vi "Main.vi"() -> ()   [LabVIEW 2015]
uses:
  TypeDefs/Queue Data.ctl
  FGV/Timer Actions.ctl
  SubVIs/App Data.vi
  SubVIs/App Strings.vi
panel:
  in  "Period [s]":dbl
  in  "Device name":tag="myDAQ1"
  out "Time Elapsed":dbl format="%<%M:%S>t"
  out "Status":string
  in  "Time [ms]":dbl
  in  "Frequency":dbl
  in  "Stop Button":bool
  in  "Acquire Button":bool
  out "Waveform Graph":dbl[](graph)
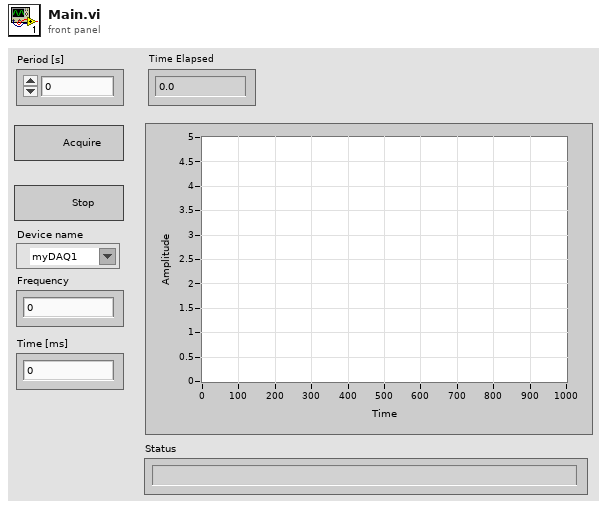
[diagram p1: front panel]
types:
  T1 = typedef "Timer Actions.ctl" = enum16{"Reset", "Get"}
  T2 = typedef "Queue Data.ctl" = cluster{"Action":string}
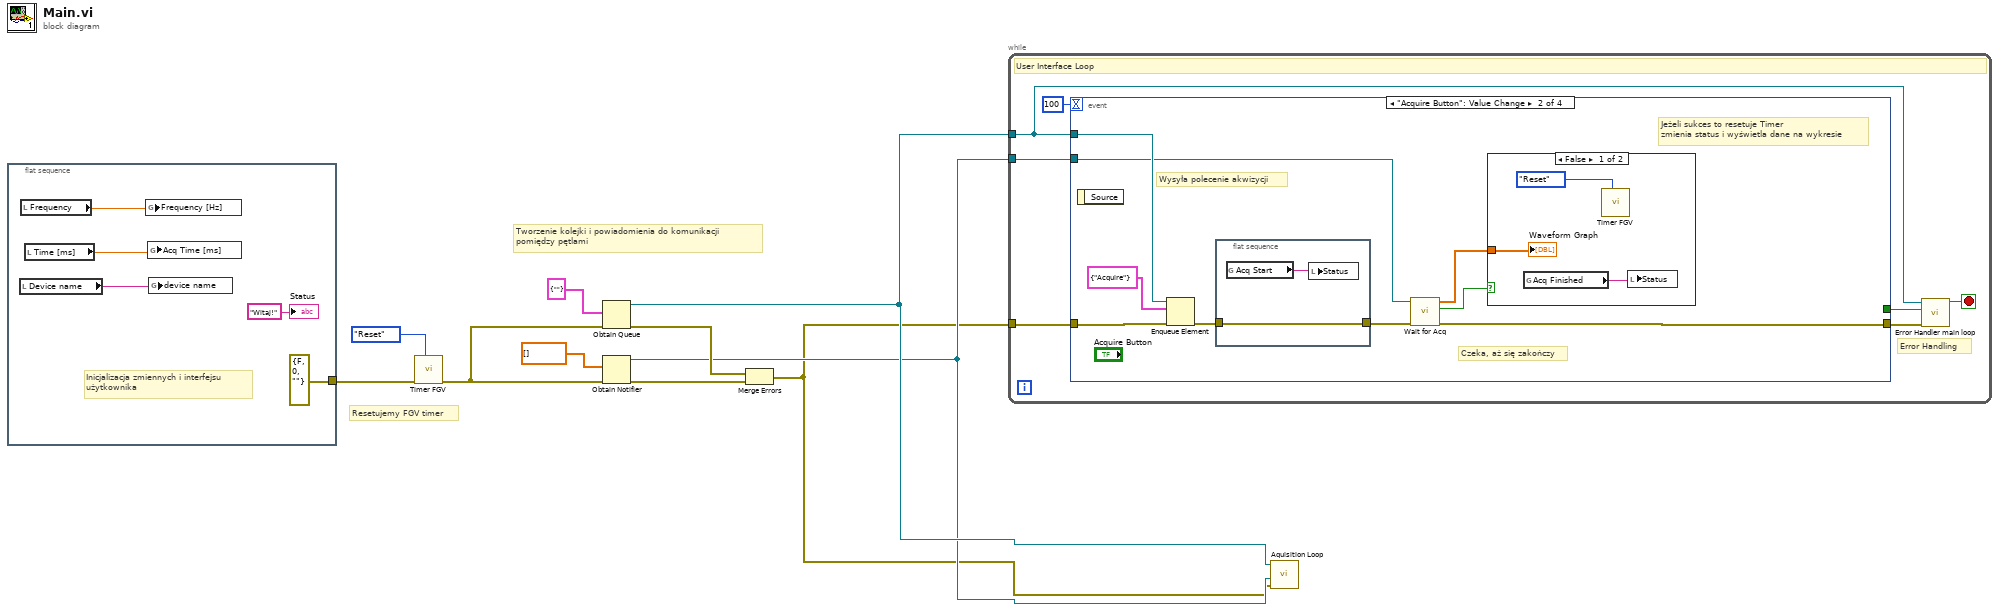
[diagram p0: block diagram]
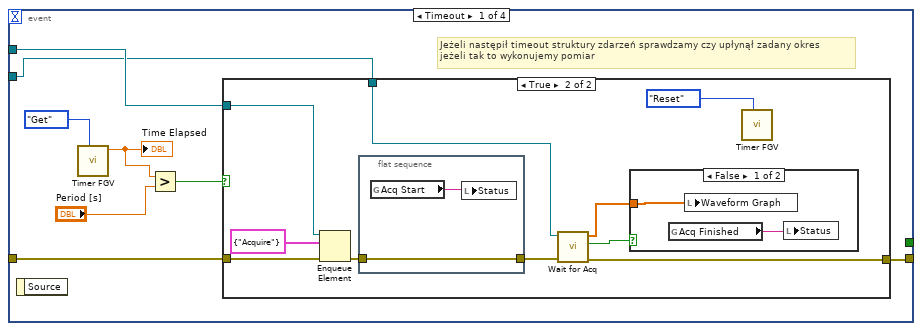
[diagram p2: hidden frame]
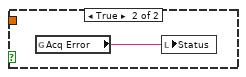
[diagram p4: hidden frame]
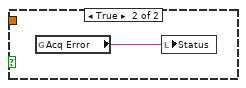
[diagram p5: hidden frame]
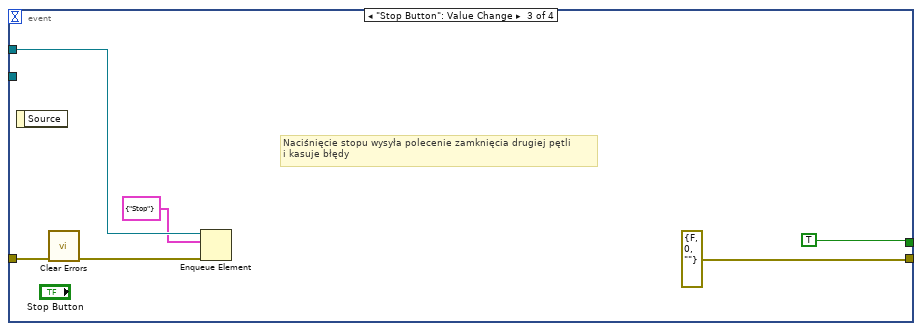
[diagram p6: hidden frame]
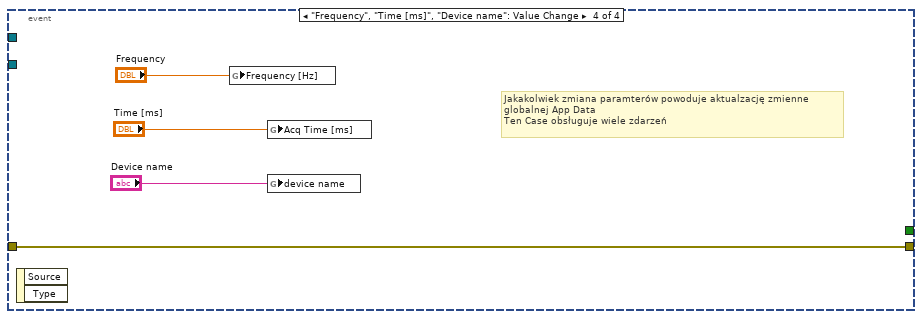
[diagram p7: hidden frame]
diagram:
  # "Resetujemy FGV timer"
  # "Tworzenie kolejki i powiadomienia do komunikacji \npomiędzy pętlami"
  n1 = flat-sequence {
    tunnel: [errorcluster {"status"=FALSE, "code"=0, "source"=""} ("error constant")] -> w6
    frame #0 {
      # "Inicjalizacja zmiennych i interfejsu \nużytkownika"
      n2 = local read "Device name"() -> (w12:tag)
      n3 = local read "Frequency"() -> (w13:dbl)
      n4 = local read "Time [ms]"() -> (w11:dbl)
      n5 = global write "App Data.vi" "Frequency [Hz]"(w13) -> ()
      n6 = global write "App Data.vi" "Acq Time [ms]"(w11) -> ()
      n7 = global write "App Data.vi" "device name"(w12) -> ()
      "Status" <- "Witaj!" ("Status")
    }
  }
  n8 = call "Timer FGV.vi"("Action"=Timer_Actions."Reset", "error in (no error)"=w6) -> ("error out"=w5:errorcluster)  [unwired: 8 in, 1 out]
  n9 = Obtain Queue(element data type=T2 {"Action"=""}, error in (no error)=w5) -> (queue out=w3:refnum<queue>, error out=w9:errorcluster)  [unwired: 3 in, 1 out]
  n10 = Obtain Notifier(notification data type=dbl[] [], error in (no error)=w5) -> (notifier out=w2:refnum<notifier>, error out=w7:errorcluster)  [unwired: 2 in, 1 out]
  n11 = Merge Errors(w9, w7) -> (w1:errorcluster)
  n12 = while {
    tunnel: w1 -> [w21]
    tunnel: w3 -> [w16]
    tunnel: w2 -> [w20]
    stop <- w17 stop-if-true
    # "Error Handling"
    # "User Interface Loop"
    n13 = event shown="[1] \"Acquire Button\": Value Change" {
      selector: _ -> [_ _ _ _]
      dyn-events: _ -> [_ _ _ _]
      timeout: 100 -> [_ _ _ _]
      tunnel: w16 -> [w25 w55 w66 _]
      tunnel: w21 -> [w26 w54 w63 w69]
      tunnel: w20 -> [w24 w52 _ _]
      tunnel: [w23 w50 errorcluster {"status"=FALSE, "code"=0, "source"=""} ("error constant") w69] -> w18
      tunnel: [_ _ TRUE _] -> w19
      event Timeout {
        # "Jeżeli następił timeout struktury zdarzeń sprawdzamy czy upłynął zadany okres \njeżeli tak to wykonujemy pomiar"
        n14 = event-data() -> ()  [unwired: 1 in, 1 out]
        n15 = call "Timer FGV.vi"("Action"=Timer_Actions."Get") -> ("Elapsed Time"=w29:dbl)  [unwired: 9 in, 1 out]
        "Time Elapsed" <- w29
        n16 = Greater?(x=w29, y="Period [s]") -> (0:w27:bool)
        n17 = case shown="True" w27 {
          tunnel: w26 -> [w31 w41]
          tunnel: w25 -> [_ w40]
          tunnel: w24 -> [_ w36]
          tunnel: [w31 w32] -> w23
          frame False {
          }
          frame True {
            n18 = Enqueue Element(queue=w40, element=T2 {"Action"="Acquire"}, error in (no error)=w41) -> (error out=w38:errorcluster)  [unwired: 1 in, 2 out]
            n19 = flat-sequence {
              tunnel: w38 -> [w45]
              tunnel: [w45] -> w37
              frame #0 {
                n20 = global read "App Strings.vi" "Acq Start"() -> (w46:string)
                n21 = local write "Status"(w46) -> ()
              }
            }
            n22 = call "Wait for Acq.vi"("error in (no error)"=w37, "Notifier in"=w36) -> ("error out"=w32:errorcluster, "timed out?"=w33:bool, "Array"=w35:dbl[])  [unwired: 7 in]
            n23 = case shown="False" w33 {
              tunnel: w35 -> [w42 _]
              frame False {
                n24 = global read "App Strings.vi" "Acq Finished"() -> (w43:string)
                n25 = local write "Waveform Graph"(w42) -> ()
                n26 = local write "Status"(w43) -> ()
              }
              frame True {
                n27 = global read "App Strings.vi" "Acq Error"() -> (w44:string)
                n28 = local write "Status"(w44) -> ()
              }
            }
            n29 = call "Timer FGV.vi"("Action"=Timer_Actions."Reset") -> ()  [unwired: 9 in, 2 out]
          }
        }
      }
      event "Acquire Button": Value Change {
        # "Jeżeli sukces to resetuje Timer\nzmienia status i wyświetla dane na wykresie"
        # "Czeka, aż się zakończy"
        # "Wysyła polecenie akwizycji"
        n30 = event-data() -> ()  [unwired: 1 in, 1 out]
        n31 = Enqueue Element(queue=w55, element=T2 {"Action"="Acquire"}, error in (no error)=w54) -> (error out=w49:errorcluster)  [unwired: 1 in, 2 out]
        n32 = flat-sequence {
          tunnel: w49 -> [w61]
          tunnel: [w61] -> w48
          frame #0 {
            n33 = global read "App Strings.vi" "Acq Start"() -> (w60:string)
            n34 = local write "Status"(w60) -> ()
          }
        }
        n35 = call "Wait for Acq.vi"("error in (no error)"=w48, "Notifier in"=w52) -> ("error out"=w50:errorcluster, "timed out?"=w47:bool, "Array"=w51:dbl[])  [unwired: 7 in]
        n36 = case shown="False" w47 {
          tunnel: w51 -> [w58 _]
          frame False {
            n37 = global read "App Strings.vi" "Acq Finished"() -> (w57:string)
            n38 = call "Timer FGV.vi"("Action"=Timer_Actions."Reset") -> ()  [unwired: 9 in, 2 out]
            n39 = local write "Status"(w57) -> ()
            "Waveform Graph" <- w58
          }
          frame True {
            n40 = global read "App Strings.vi" "Acq Error"() -> (w59:string)
            n41 = local write "Status"(w59) -> ()
          }
        }
      }
      event "Stop Button": Value Change {
        # "Naciśnięcie stopu wysyła polecenie zamknięcia drugiej pętli\ni kasuje błędy"
        n42 = event-data() -> ()  [unwired: 1 in, 1 out]
        n43 = call <vilib>:"Clear Errors.vi"("error in (no error)"=w63) -> ("error out"=w62:errorcluster)  [unwired: 5 in, 1 out]
        n44 = Enqueue Element(queue=w66, element=T2 {"Action"="Stop"}, error in (no error)=w62) -> ()  [unwired: 1 in, 3 out]
      }
      event "Frequency", "Time [ms]", "Device name": Value Change {
        # "Jakakolwiek zmiana paramterów powoduje aktualzację zmienne \nglobalnej App Data\nTen Case obsługuje wiele zdarzeń"
        n45 = event-data() -> ()  [unwired: 1 in, 2 out]
        n46 = global write "App Data.vi" "Frequency [Hz]"("Frequency") -> ()
        n47 = global write "App Data.vi" "Acq Time [ms]"("Time [ms]") -> ()
        n48 = global write "App Data.vi" "device name"("Device name") -> ()
      }
    }
    n49 = call "Error Handler main loop.vi"("error in (no error)"=w18, "Exit?"=w19, "Queue in"=w16) -> ("Exit?"=w17:bool)  [unwired: 8 in]
  }
  n50 = call "Aquisition Loop.vi"("error out"=w1, "notifier out"=w2, "queue out"=w3) -> ()  [unwired: 9 in]
